vi "WPI_CameraSet Brightness.vi"(6 "Force":bool, 8 "error in (no error)":errorcluster, 10 "Brightness":i32=50 min=0 max=100, 11 "CameraDevRef":T1={"Camera Address"="192.168.0.90", "CameraStatus"={"status"=FALSE, "code"=0, "source"=""}}) -> (0 "error out":errorcluster, 3 "CameraDevRef Out":T1)   [LabVIEW 2017]
doc: "Specifies the brightness setting of the camera you specify.\n\nThis software is licensed. Open the labview\\readme\\WPI Robotics Library Open Source License.txt file for more information."
uses:
  <vilib>/Rock Robotics/WPI/Camera/WPI_CameraDevRef.ctl
  <vilib>/Rock Robotics/WPI/Camera/WPI_CameraSettings Operations.ctl
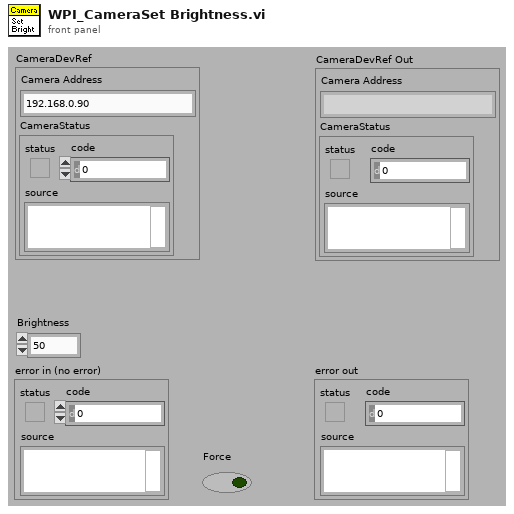
[diagram p1: front panel]
types:
  T1 = typedef "WPI_CameraDevRef.ctl" = cluster{"Camera Address":string, "CameraStatus":errorcluster}
  T2 = typedef "WPI_CameraSettings Operations.ctl" = enum16{"Udate FPS", "Update Compression", "Update Size", "Update White Balance", "Update Brightness", "Update Sharpness", "Update Exposure", "Update Exposure Value", "Update Color Level", "Update Exp Priority", "Update Color Enable", "Update JPG", "Update MJPG", "Read and Clear", "Read", "Init"}
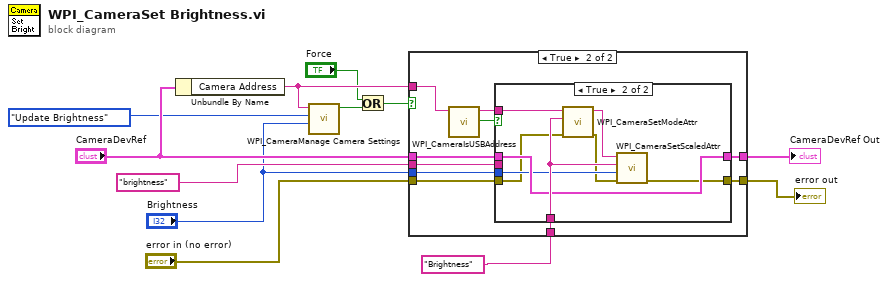
[diagram p0: block diagram]
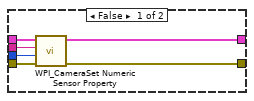
[diagram p3: hidden frame]
diagram:
  n1 = Unbundle By Name("CameraDevRef") -> ("Camera Address"=w5:string)
  n2 = call <vilib>:"WPI_CameraManage Camera Settings.vi"("Value"="Brightness", "Operation"=WPI_CameraSettings_Operations."Update Brightness", "Camera IP"=w5) -> ("Changed"=w2:bool)  [unwired: 7 in, 1 out]
  n3 = Or(x="Force", y=w2) -> (x .or. y?=w1:bool)
  n4 = case shown="True" w1 {
    tunnel: "brightness" ("Property Name") -> [_ w24]
    tunnel: [w14 w23] -> w11
    tunnel: "error in (no error)" -> [w13 w22]
    tunnel: [w13 w21] -> w9
    tunnel: "CameraDevRef" -> [w14 w20]
    tunnel: "Brightness" -> [_ w19]
    tunnel: w5 -> [_ w16]
    tunnel: "Brightness" -> [_ w15]
    frame False {
    }
    frame True {
      n5 = call <vilib>:"WPI_CameraIsUSBAddress.vi"("Camera Address In"=w16) -> ("USB?"=w18:bool, "Camera Address Out"=w17:string)  [unwired: 8 in, 1 out]
      n6 = case shown="True" w18 {
        tunnel: w24 -> [w30 _]
        tunnel: [w29 w35] -> w23
        tunnel: w22 -> [w28 w32]
        tunnel: [w27 w31] -> w21
        tunnel: w20 -> [w26 w35]
        tunnel: w19 -> [w25 w34]
        tunnel: w17 -> [_ w36]
        tunnel: w15 -> [_ w37]
        frame False {
          n7 = call <vilib>:"WPI_CameraSet Numeric Sensor Property.vi"("error in (no error)"=w28, "Value"=w25, "Property Name"=w30, "CameraDevRef"=w26) -> ("error out"=w27:errorcluster, "CameraDevRef out"=w29:T1)  [unwired: 4 in, 2 out]
        }
        frame True {
          n8 = call <vilib>:"WPI_CameraSetModeAttr.vi"("error in (no error)"=w32, "Attr String"=w37, "Camera Address In"=w36) -> ("error out"=w33:errorcluster, "Camera Address Out"=w38:string)  [unwired: 7 in]
          n9 = call <vilib>:"WPI_CameraSetScaledAttr.vi"("error in (no error)"=w33, "Scaled"=w34, "Attr String"=w37, "Camera Address In"=w38) -> ("error out"=w31:errorcluster)  [unwired: 6 in, 1 out]
        }
      }
    }
  }
  "CameraDevRef Out" <- w11
  "error out" <- w9
